vi "读取历史数据.vi"() -> ()   [LabVIEW 2018]
panel:
  out "基本数据":string[][](array[string])
  out "光谱":dbl[](graph)
  out "远场":T1(plugin-control)
  out "近场":T1(plugin-control)
  out "时间波形":dbl[](graph)
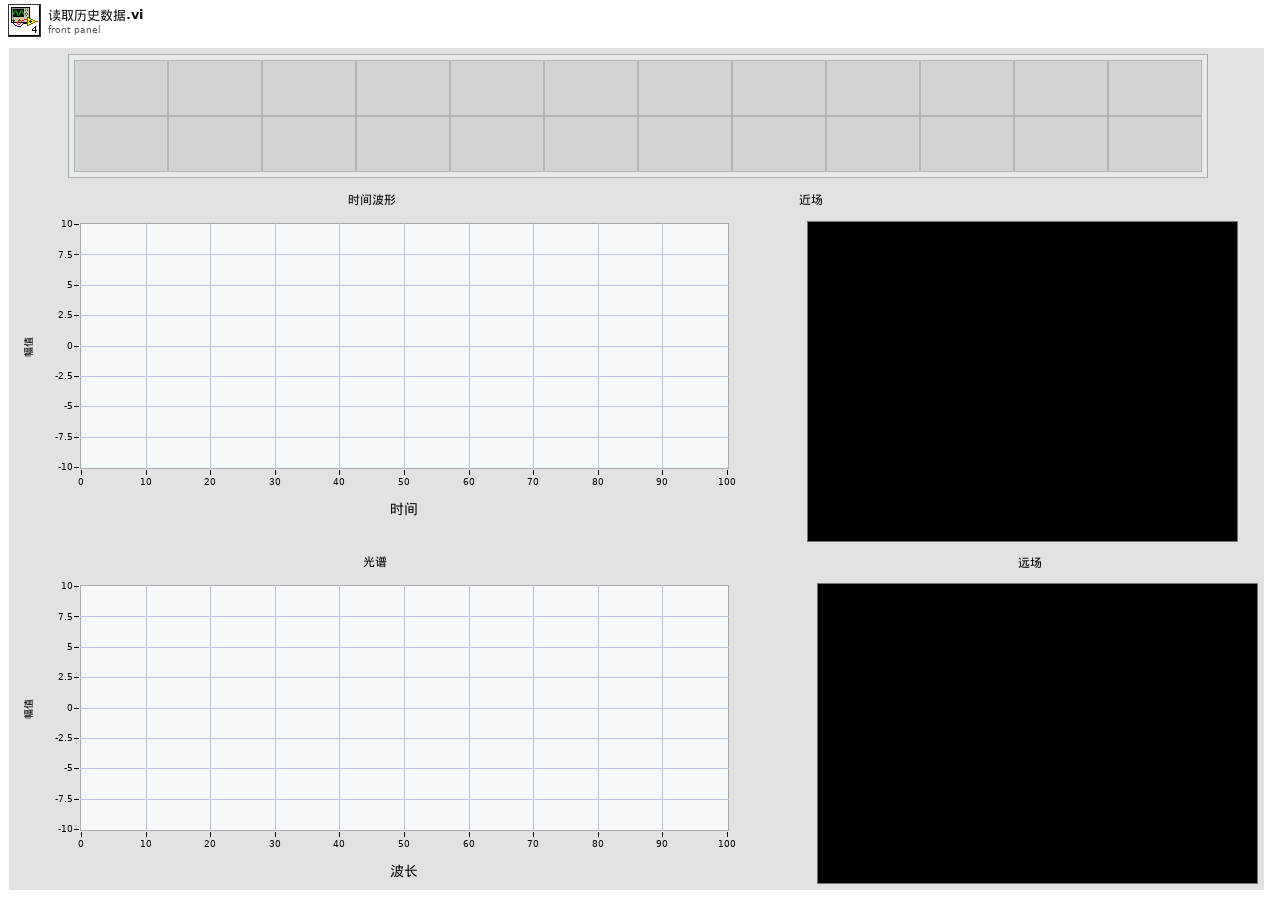
[diagram p1: front panel]
types:
  T1 = typedef "IMAQ Image.ctl" = refnum<image>
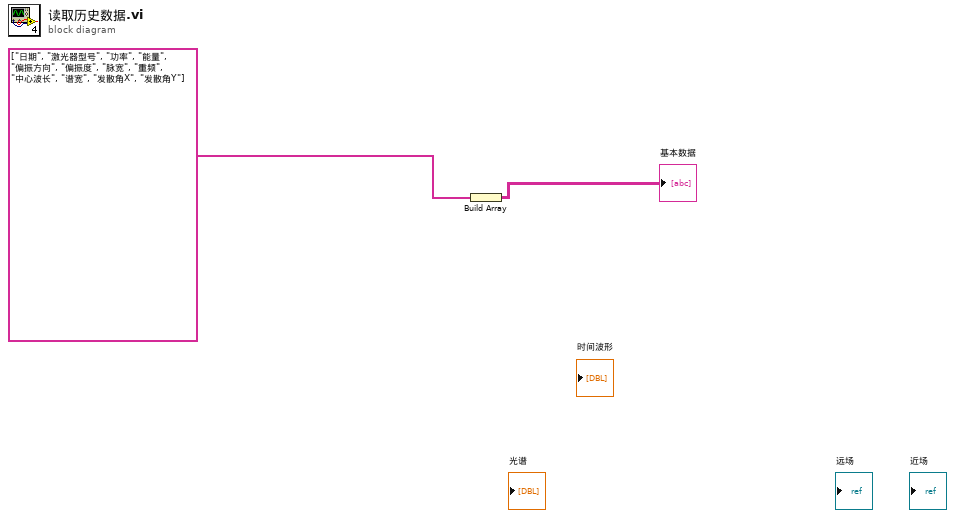
[diagram p0: block diagram]
diagram:
  n1 = Build Array(string[] ["日期", "激光器型号", "功率", "能量", "偏振方向", "偏振度", "脉宽", "重频", "中心波长", "谱宽", "发散角X", "发散角Y"]) -> (→"基本数据":string[][])
